vi "Load by Identifier.vi"(8 "error in (no error)":errorcluster, 10 "Identifier":string, 11 "User DB in":refnum<class "User DB.lvclass">) -> (0 "error out":errorcluster, 2 "User":refnum<class "User.lvclass">, 3 "User DB out":refnum<class "User DB.lvclass">)   [LabVIEW 2020, in "Summer of LabVIEW.lvlib" / "User DB.lvclass"]
uses:
  User DB.lvclass
  <vilib>/IlluminatedG/IG HTTP Server/HTTP Server/User/User.lvclass
  User DB.lvclass/User DB.ctl
  <vilib>/drjdpowell/SQLite Library/SQL Statement/SQL Statement.lvclass/SQL Statement.ctl
  SOL User/User Data.ctl
  <vilib>/drjdpowell/SQLite Library/SQL Statement/Column I64.vi
  <vilib>/drjdpowell/SQLite Library/SQL Statement/Bind Text.vi
  <vilib>/drjdpowell/SQLite Library/SQL Statement/Step.vi
  SOL User/SOL User.lvclass
  C:/Program Files (x86)/National Instruments/LabVIEW 2020/vi.lib/IlluminatedG/IG HTTP Server/HTTP Server/User/User.lvclass
  <vilib>/drjdpowell/SQLite Library/SQL Statement/Error Message.vi
  <vilib>/drjdpowell/SQLite Library/SQL Statement/Column String.vi
  SQLite/SQLite.lvclass
  <vilib>/drjdpowell/SQLite Library/SQL Connection/Connection.lvclass
  <vilib>/drjdpowell/SQLite Library/SQL Statement/SQL Statement.lvclass
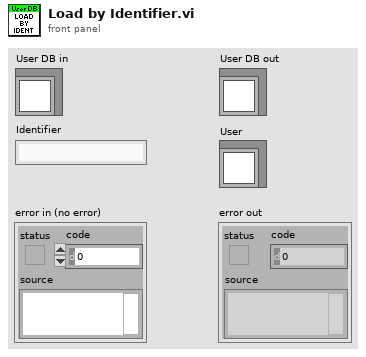
[diagram p1: front panel]
types:
  T1 = typedef "Summer of LabVIEW.lvlib/SOL User.lvclass/User Data.ctl" = cluster{"ID":i64, "Email":string, "Encoded Password":string, "Roles":string[], "First Name":string, "Last Name":string, "Department":string}
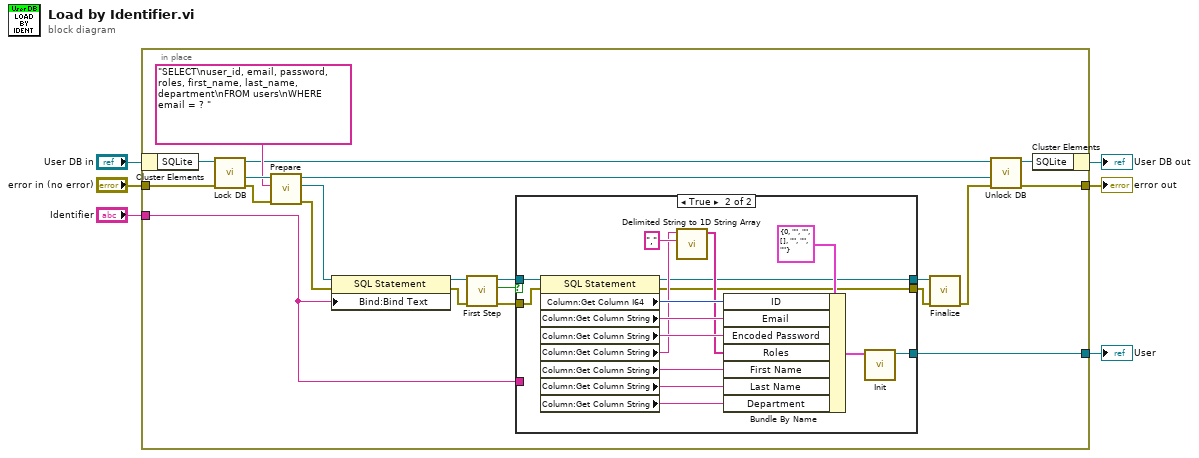
[diagram p0: block diagram]
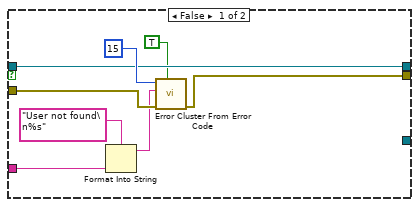
[diagram p2: hidden frame]
diagram:
  n1 = in-place {
    in-place-border: "error in (no error)" -> [w27]
    in-place-border: "Identifier" -> [w14]
    in-place-border: [w15] -> w1
    in-place-border: [w10] -> w3
    n2 = in-place-cluster #1("User DB in") -> ("SQLite"=w26:refnum<class "SQLite.lvclass">)
    n3 = call "Lock DB.vi"("error in (no error)"=w27, "SQLite in"=w26) -> ("error out"=w24:errorcluster, "SQLite DB"=w25:refnum<class "Connection.lvclass">, "SQLite out"=w12:refnum<class "SQLite.lvclass">)  [unwired: 6 in, 1 out]
    n4 = call <vilib>:"Prepare.vi"("error in (no error)"=w24, "SQL"="SELECT\nuser_id, email, password, roles, first_name, last_name, department\nFROM users\nWHERE email = ? ", "SQLite Connection in"=w25) -> ("error out"=w22:errorcluster, "SQL Statement"=w21:refnum<class "SQL Statement.lvclass">, "SQLite Connection"=w11:refnum<class "Connection.lvclass">)  [unwired: 4 in, 2 out]
    n5 = property class="SQL Statement"(reference=w21, error in=w22, "Bind:Bind Text"=w14) -> (reference out=w19:refnum<class "SQL Statement.lvclass">, error out=w20:errorcluster)
    n6 = call <vilib>:"First Step.vi"("error in (no error)"=w20, "SQL Statement in"=w19) -> ("error out"=w18:errorcluster, "Row returned"=w17:bool, "SQL Statement"=w16:refnum<class "SQL Statement.lvclass">)  [unwired: 7 in]
    n7 = case shown="True" w17 {
      tunnel: w18 -> [w34 w50]
      tunnel: w16 -> [w29 w51]
      tunnel: [_ w38] -> w15
      tunnel: w14 -> [w32 _]
      tunnel: [w30 w37] -> w9
      tunnel: [w29 w36] -> w8
      frame False {
        n8 = Format Into String(format string="User not found\n%s", w32) -> (resulting string=w31:string)  [unwired: 2 in, 1 out]
        n9 = call <vilib>:"Error Cluster From Error Code.vi"("show call chain? (False)"=TRUE, "error in (no error)"=w34, "error message (\"\")"=w31, "error code (0)"=15) -> ("error out"=w30:errorcluster)  [unwired: 5 in]
      }
      frame True {
        n10 = property on="Extract Column Data" class="SQL Statement"(reference=w51, error in=w50) -> (reference out=w36:refnum<class "SQL Statement.lvclass">, error out=w37:errorcluster, "Column:Get Column I64"=w42:i64, "Column:Get Column String"=w43:string, "Column:Get Column String"=w44:string, "Column:Get Column String"=w40:string, "Column:Get Column String"=w45:string, "Column:Get Column String"=w46:string, "Column:Get Column String"=w47:string)
        n11 = call <vilib>:"Delimited String to 1D String Array.vi"("delimiter"=",", "delimited string"=w40) -> ("string array"=w39:string[])  [unwired: 9 in]
        n12 = Bundle By Name(cluster=T1 {"ID"=0, "Email"="", "Encoded Password"="", "Roles"=[], "First Name"="", "Last Name"="", "Department"=""} ("User Data"), "ID"=w42, "Email"=w43, "Encoded Password"=w44, "Roles"=w39, "First Name"=w45, "Last Name"=w46, "Department"=w47) -> (w48:T1)
        n13 = call "Init.vi"("User Data"=w48) -> ("SOL User out"=w38:refnum<class "SOL User.lvclass">)  [unwired: 9 in, 1 out]
      }
    }
    n14 = call <vilib>:"Finalize.vi"("error in (no error)"=w9, "SQL Statement in"=w8) -> ("error out"=w7:errorcluster)  [unwired: 9 in]
    n15 = call "Unlock DB.vi"("error in (no error)"=w7, "SQLite DB"=w11, "SQLite in"=w12) -> ("error out"=w10:errorcluster, "SQLite out"=w13:refnum<class "SQLite.lvclass">)  [unwired: 7 in]
    n16 = in-place-cluster #1("SQLite"=w13) -> (→"User DB out":refnum<class "User DB.lvclass">)
  }
  "error out" <- w3
  "User" <- w1
